vi "Test Set Subpanels-- SMO Array -- Started -- Unique.vi"(8 "error in":errorcluster) -> (0 "error out":errorcluster)   [LabVIEW 2020]
uses:
  Maui 2.0/Maui 2.0.lvclass
  C:/Program Files (x86)/National Instruments/LabVIEW 2020/vi.lib/JKI/JKI SMO/SMO/SMO.lvclass
  <vilib>/addons/_JKI Toolkits/Caraya/classes/Assert/Assert True.vi
  <vilib>/addons/_JKI Toolkits/Caraya/classes/Assert/Assert Equal Value_Variant.vi
  <vilib>/addons/_JKI Toolkits/Caraya/classes/Test/Test.lvclass
  <vilib>/JKI/JKI SMO/SMO/SMO.lvclass
  <vilib>/addons/_JKI Toolkits/Caraya/classes/Assert/Assert.lvclass
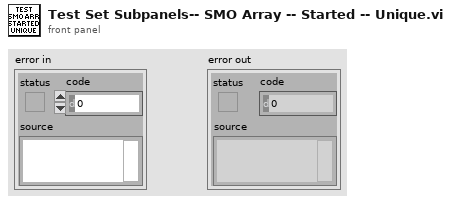
[diagram p1: front panel]
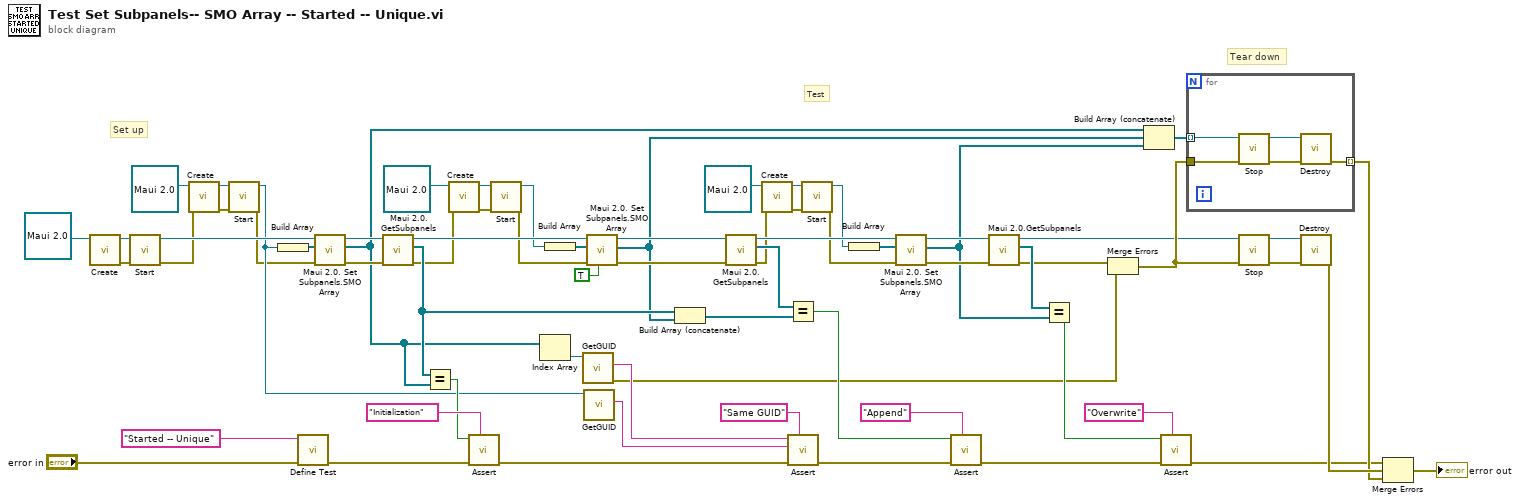
[diagram p0: block diagram]
diagram:
  # "Tear down"
  # "Test"
  # "Set up"
  n1 = call <vilib>:"Create.vi"("SMO"=refnum<class "Maui 2.0.lvclass"> refnum ("Maui 2.0.lvclass")) -> ("error out"=w64:errorcluster, "SMO out"=w63:refnum<class "Maui 2.0.lvclass">)  [unwired: 8 in, 1 out]
  n2 = call <vilib>:"Start.vi"("error in (no error)"=w64, "SMO"=w63) -> ("error out"=w3:errorcluster, "SMO out"=w61:refnum<class "Maui 2.0.lvclass">)  [unwired: 8 in]
  n3 = call <vilib>:"Create.vi"("error in (no error)"=w3, "SMO"=refnum<class "Maui 2.0.lvclass"> refnum ("Maui 2.0.lvclass")) -> ("error out"=w1:errorcluster, "SMO out"=w23:refnum<class "Maui 2.0.lvclass">)  [unwired: 7 in, 1 out]
  n4 = call <vilib>:"Start.vi"("error in (no error)"=w1, "SMO"=w23) -> ("error out"=w2:errorcluster, "SMO out"=w10:refnum<class "Maui 2.0.lvclass">)  [unwired: 8 in]
  n5 = Build Array(w10) -> (w25:refnum<class "Maui 2.0.lvclass">[])
  n6 = call <vilib>:"Define Test.vi"("error in (no error)"="error in", "Label (VI Title)"="Started -- Unique") -> ("error out"=w67:errorcluster)  [unwired: 9 in]
  n7 = call-dynamic "Maui 2.0. Set Subpanels.SMO Array.vi"("error in (no error)"=w2, "Subpanels"=w25, "Maui 2.0 in"=w61) -> ("error out"=w54:errorcluster, "Subpanels"=w42:refnum<class "SMO.lvclass">[], "Maui 2.0 out"=w55:refnum<class "Maui 2.0.lvclass">)  [unwired: 6 in]
  n8 = call "Maui 2.0.GetSubpanels.vi"("error in (no error)"=w54, "Maui 2.0"=w55) -> ("error out"=w8:errorcluster, "Subpanels"=w43:refnum<class "SMO.lvclass">[], "Maui 2.0 out"=w44:refnum<class "Maui 2.0.lvclass">)  [unwired: 7 in]
  n9 = Equal?(x=w43, y=w42) -> (x = y?=w41:bool)
  n10 = call <vilib>:"Create.vi"("error in (no error)"=w8, "SMO"=refnum<class "Maui 2.0.lvclass"> refnum ("Maui 2.0.lvclass")) -> ("error out"=w9:errorcluster, "SMO out"=w22:refnum<class "Maui 2.0.lvclass">)  [unwired: 7 in, 1 out]
  n11 = call-poly <vilib>:"Assert.vi"("Label"="Initialization", "error in (no error)"=w67, "True?"=w41) -> ("error out"=w51:errorcluster)  [unwired: 8 in]
  n12 = call <vilib>:"Start.vi"("error in (no error)"=w9, "SMO"=w22) -> ("error out"=w7:errorcluster, "SMO out"=w11:refnum<class "Maui 2.0.lvclass">)  [unwired: 8 in]
  n13 = Index Array(array=w42) -> (element=w16:refnum<class "SMO.lvclass">)  [unwired: 1 in]
  n14 = Build Array(w11) -> (w12:refnum<class "Maui 2.0.lvclass">[])
  n15 = call <vilib>:"GetGUID.vi"("SMO"=w16) -> ("error out"=w13:errorcluster, "GUID"=w15:string)  [unwired: 8 in, 1 out]
  n16 = call <vilib>:"GetGUID.vi"("SMO"=w10) -> ("GUID"=w14:string)  [unwired: 8 in, 2 out]
  n17 = call-dynamic "Maui 2.0. Set Subpanels.SMO Array.vi"("Append (F)"=TRUE, "error in (no error)"=w7, "Subpanels"=w12, "Maui 2.0 in"=w44) -> ("error out"=w46:errorcluster, "Subpanels"=w37:refnum<class "SMO.lvclass">[], "Maui 2.0 out"=w45:refnum<class "Maui 2.0.lvclass">)  [unwired: 5 in]
  n18 = Build Array (concatenate)(w43, w37) -> (w39:refnum<class "SMO.lvclass">[])
  n19 = call "Maui 2.0.GetSubpanels.vi"("error in (no error)"=w46, "Maui 2.0"=w45) -> ("error out"=w5:errorcluster, "Subpanels"=w40:refnum<class "SMO.lvclass">[], "Maui 2.0 out"=w31:refnum<class "Maui 2.0.lvclass">)  [unwired: 7 in]
  n20 = call <vilib>:"Create.vi"("error in (no error)"=w5, "SMO"=refnum<class "Maui 2.0.lvclass"> refnum ("Maui 2.0.lvclass")) -> ("error out"=w6:errorcluster, "SMO out"=w19:refnum<class "Maui 2.0.lvclass">)  [unwired: 7 in, 1 out]
  n21 = Equal?(x=w40, y=w39) -> (x = y?=w26:bool)
  n22 = call-poly <vilib>:"Assert.vi"("Label"="Same GUID", "error in (no error)"=w51, "Y"=w14, "X"=w15) -> ("error out"=w52:errorcluster)  [unwired: 7 in]
  n23 = call <vilib>:"Start.vi"("error in (no error)"=w6, "SMO"=w19) -> ("error out"=w4:errorcluster, "SMO out"=w18:refnum<class "Maui 2.0.lvclass">)  [unwired: 8 in]
  n24 = Build Array(w18) -> (w17:refnum<class "Maui 2.0.lvclass">[])
  n25 = call-dynamic "Maui 2.0. Set Subpanels.SMO Array.vi"("error in (no error)"=w4, "Subpanels"=w17, "Maui 2.0 in"=w31) -> ("error out"=w34:errorcluster, "Subpanels"=w27:refnum<class "SMO.lvclass">[], "Maui 2.0 out"=w35:refnum<class "Maui 2.0.lvclass">)  [unwired: 6 in]
  n26 = call-poly <vilib>:"Assert.vi"("Label"="Append", "error in (no error)"=w52, "True?"=w26) -> ("error out"=w48:errorcluster)  [unwired: 8 in]
  n27 = call "Maui 2.0.GetSubpanels.vi"("error in (no error)"=w34, "Maui 2.0"=w35) -> ("error out"=w32:errorcluster, "Subpanels"=w33:refnum<class "SMO.lvclass">[], "Maui 2.0 out"=w30:refnum<class "Maui 2.0.lvclass">)  [unwired: 7 in]
  n28 = Equal?(x=w33, y=w27) -> (x = y?=w29:bool)
  n29 = Merge Errors(w32, w13) -> (w50:errorcluster)
  n30 = Build Array (concatenate)(w42, w37, w27) -> (w57:refnum<class "SMO.lvclass">[])
  n31 = call-poly <vilib>:"Assert.vi"("Label"="Overwrite", "error in (no error)"=w48, "True?"=w29) -> ("error out"=w47:errorcluster)  [unwired: 8 in]
  n32 = for {
    tunnel: w57 -> [w71] mode=indexing
    tunnel: w50 -> [w70]
    tunnel: [w69] -> w56 mode=indexing
    n33 = call <vilib>:"Stop.vi"("error in (no error)"=w70, "SMO"=w71) -> ("error out"=w72:errorcluster, "SMO out"=w73:refnum<class "SMO.lvclass">)  [unwired: 8 in]
    n34 = call <vilib>:"Destroy.vi"("error in (no error)"=w72, "SMO"=w73) -> ("error out"=w69:errorcluster)  [unwired: 9 in]
  }
  n35 = call <vilib>:"Stop.vi"("error in (no error)"=w50, "SMO"=w30) -> ("error out"=w60:errorcluster, "SMO out"=w59:refnum<class "Maui 2.0.lvclass">)  [unwired: 8 in]
  n36 = call <vilib>:"Destroy.vi"("error in (no error)"=w60, "SMO"=w59) -> ("error out"=w58:errorcluster)  [unwired: 9 in]
  n37 = Merge Errors(w47, w58, w56) -> (→"error out":errorcluster)
